vi "SubVI_Resize_Grayscale_Image #.vi"(5 "Image Register Name":string="untitled", 7 "Magnification":i32 min=1 max=9 step=1, 8 "Error In":errorcluster, 10 "ROI Descriptor":T2 {"Contours"."Type" items=["No Selection", "Point", "Line", "Rectangle", "Oval", "Polygon", "Freehand Region", "Annulus", "Unused2", "Unused3", "Broken Line", "Freehand Line", "Rotated Rectangle"]}, 11 "Image Src In":T1) -> (0 "Error Out":errorcluster, 1 "Image Src Out":T1, 2 "ROI Descriptor out":T2 {"Contours"."Type" items=["No Selection", "Point", "Line", "Rectangle", "Oval", "Polygon", "Freehand Region", "Annulus", "Unused2", "Unused3", "Broken Line", "Freehand Line", "Rotated Rectangle"]}, 3 "Image Dst Out":T1)   [LabVIEW 2013]
uses:
  <vilib>/vision/Image Controls.llb/IMAQ Image.ctl
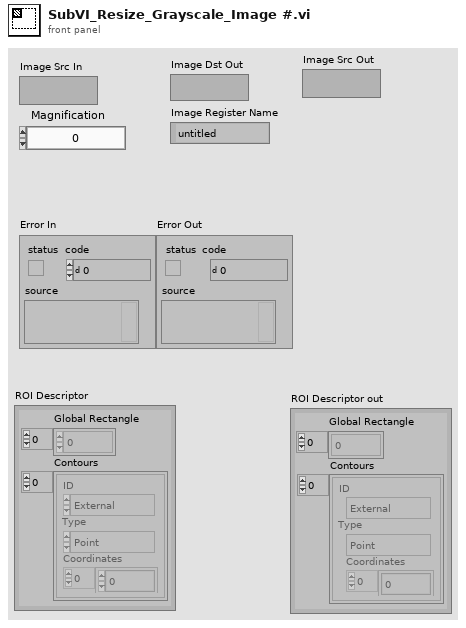
[diagram p1: front panel]
types:
  T1 = typedef "IMAQ Image.ctl" = refnum<image>
  T2 = typedef "ROI Descriptor" = cluster{"Global Rectangle":i32[], "Contours":cluster{"ID":enum32{"External", "Internal"}, "Type":u32, "Coordinates":i32[]}[]}
  T3 = enum16{"No Selection", "Point", "Line", "Rectangle", "Oval", "Polygon", "Freehand Region", "Annulus", "Unused2", "Unused3", "Broken Line", "Freehand Line", "Rotated Rectangle"}
  T4 = cluster{"ID":enum32{"External", "Internal"}, "Type":u32, "Coordinates":i32[]}[]
  T5 = cluster{"ID":enum32{"External", "Internal"}, "Type":u32, "Coordinates":i32[]}
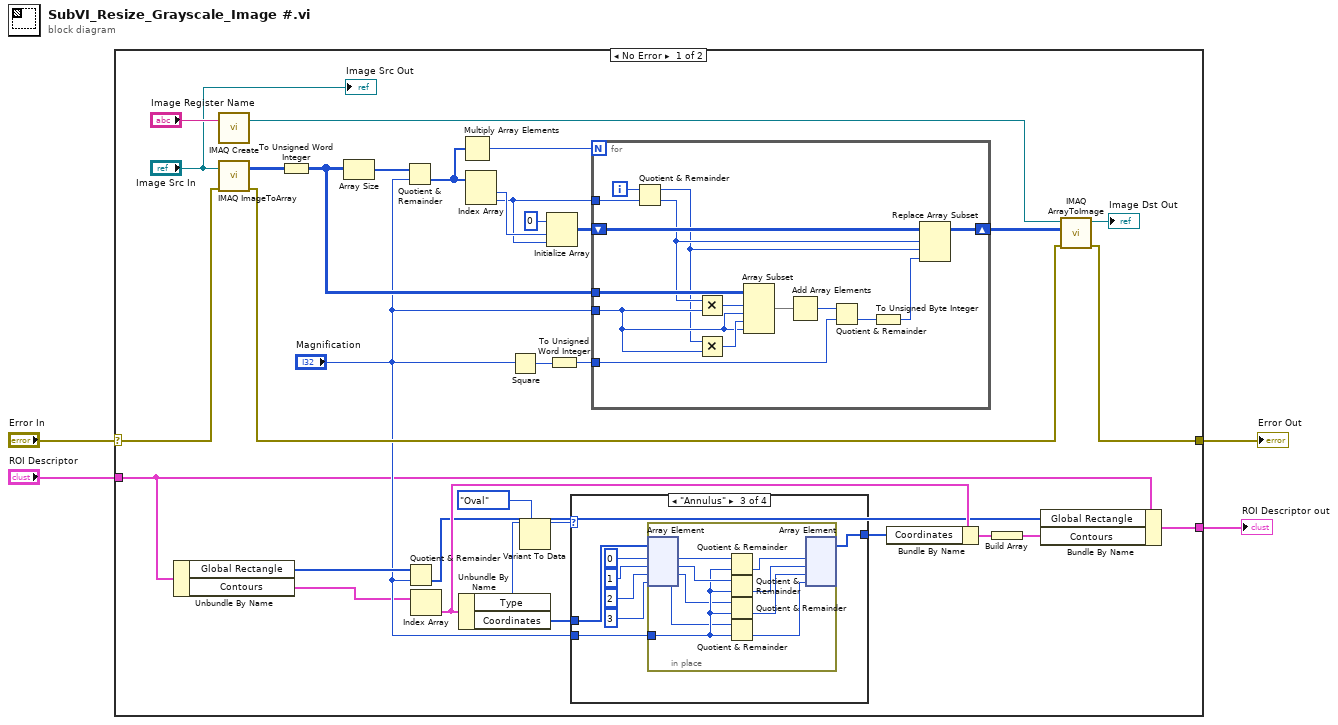
[diagram p0: block diagram]
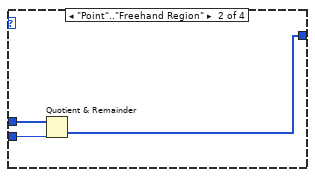
[diagram p3: hidden frame]
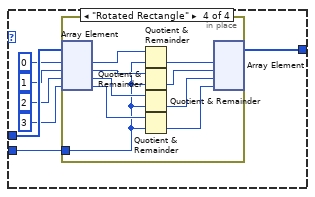
[diagram p4: hidden frame]
diagram:
  n1 = case shown="No Error" "Error In" {
    selector: "Error In" -> [w26 w90]
    tunnel: [w23 w90] -> w3
    tunnel: "ROI Descriptor" -> [w9 w89]
    tunnel: [w7 w89] -> w1
    frame No Error {
      n2 = Unbundle By Name(w9) -> ("Global Rectangle"=w19:i32[], "Contours"=w13:T4)
      n3 = call "IMAQ Create"("Image Name"="Image Register Name") -> ("New Image"=w20:T1)  [unwired: 4 in, 1 out]
      n4 = call "IMAQ ImageToArray"("error in (no error)"=w26, "Image"="Image Src In") -> ("error out"=w24:errorcluster, "Image Pixels (U8)"=w28:u8[][])  [unwired: 2 in, 3 out]
      n5 = To Unsigned Word Integer(number=w28) -> (unsigned 16bit integer=w27:u16[][])
      n6 = Array Size(array=w27) -> (size(s)=w36:i32[])
      n7 = Quotient & Remainder(x=w36, y="Magnification") -> (floor(x/y)=w37:i32[])  [unwired: 1 out]
      n8 = Quotient & Remainder(x=w19, y="Magnification") -> (floor(x/y)=w6:i32[])  [unwired: 1 out]
      n9 = Index Array(array=w13) -> (element=w12:T5)  [unwired: 1 in]
      n10 = Unbundle By Name(w12) -> ("Type"=w17:u32, "Coordinates"=w16:i32[])
      n11 = Multiply Array Elements(1:w37) -> (0:w35:i32)
      n12 = Index Array(array=w37) -> (element #1=w32:i32, element #2=w31:i32)  [unwired: 2 in]
      n13 = Square(x="Magnification") -> (x^2=w30:i32)
      n14 = Variant To Data(type=T3."Oval" ("Type"), Variant=w17) -> (data=w15:T3)  [unwired: 1 in, 1 out]
      n15 = Initialize Array(u8 0 ("element"), w32, w31) -> (w33:u8[][])
      n16 = To Unsigned Word Integer(number=w30) -> (unsigned 16bit integer=w29:u16)
      n17 = case shown="\"Annulus\"" w15 {
        tunnel: w16 -> [w38 w41 w48 w64]
        tunnel: "Magnification" -> [_ w40 w47 w63]
        tunnel: [w38 w39 w46 w62] -> w11
        frame "No Selection", Default {
        }
        frame "Point".."Freehand Region" {
          n18 = Quotient & Remainder(x=w41, y=w40) -> (floor(x/y)=w39:i32[])  [unwired: 1 out]
        }
        frame "Annulus" {
          n19 = in-place {
            in-place-border: w47 -> [w51]
            n20 = in-place-array #1(w48, 0, 1, 2, 3) -> (w57:i32, w56:i32, w50:i32, w49:i32)
            n21 = Quotient & Remainder(x=w57, y=w51) -> (floor(x/y)=w55:i32)  [unwired: 1 out]
            n22 = Quotient & Remainder(x=w56, y=w51) -> (floor(x/y)=w54:i32)  [unwired: 1 out]
            n23 = Quotient & Remainder(x=w50, y=w51) -> (floor(x/y)=w53:i32)  [unwired: 1 out]
            n24 = Quotient & Remainder(x=w49, y=w51) -> (floor(x/y)=w52:i32)  [unwired: 1 out]
            n25 = in-place-array #1(w55, w54, w53, w52) -> (w46:i32[])  [unwired: 4 out]
          }
        }
        frame "Rotated Rectangle" {
          n26 = in-place {
            in-place-border: w63 -> [w65]
            n27 = in-place-array #2(w64, 0, 1, 2, 3) -> (w69:i32, w68:i32, w67:i32, w66:i32)
            n28 = Quotient & Remainder(x=w69, y=w65) -> (floor(x/y)=w73:i32)  [unwired: 1 out]
            n29 = Quotient & Remainder(x=w68, y=w65) -> (floor(x/y)=w72:i32)  [unwired: 1 out]
            n30 = Quotient & Remainder(x=w67, y=w65) -> (floor(x/y)=w71:i32)  [unwired: 1 out]
            n31 = Quotient & Remainder(x=w66, y=w65) -> (floor(x/y)=w70:i32)  [unwired: 1 out]
            n32 = in-place-array #2(w73, w72, w71, w70) -> (w62:i32[])  [unwired: 4 out]
          }
        }
      }
      n33 = for {
        N: w35 -> [_]
        shift-right: [w74] -> w25
        shift-left: w33 -> [w78]
        tunnel: w31 -> [w87]
        tunnel: w27 -> [w81]
        tunnel: w29 -> [w80]
        tunnel: "Magnification" -> [w79]
        i -> [w88]
        n34 = Quotient & Remainder(x=w88, y=w87) -> (x-y*floor(x/y)=w75:i32, floor(x/y)=w76:i32)
        n35 = Multiply(x=w76, y=w79) -> (x*y=w83:i32)
        n36 = Multiply(x=w75, y=w79) -> (x*y=w84:i32)
        n37 = Array Subset(array=w81, index (row)=w83, length (row)=w79, index (col)=w84, length (col)=w79) -> (w82:u16[][])
        n38 = Add Array Elements(numeric array=w82) -> (sum=w86:u16)
        n39 = Quotient & Remainder(x=w86, y=w80) -> (floor(x/y)=w85:u16)  [unwired: 1 out]
        n40 = To Unsigned Byte Integer(number=w85) -> (unsigned 8bit integer=w77:u8)
        n41 = Replace Array Subset(array=w78, new element=w77, index (row)=w76, index (col)=w75) -> (w74:u8[][])
      }
      n42 = Bundle By Name(cluster=w12, "Coordinates"=w11) -> (w10:T5)
      n43 = Build Array(w10) -> (w8:T4)
      n44 = Bundle By Name(cluster=w9, "Global Rectangle"=w6, "Contours"=w8) -> (w7:T2)
      n45 = call "IMAQ ArrayToImage"("error in (no error)"=w24, "Image Pixels (U8)"=w25, "Image"=w20) -> ("error out"=w23:errorcluster, "Image Out"=→"Image Dst Out":T1)  [unwired: 7 in]
      "Image Src Out" <- "Image Src In"
    }
    frame Error {
    }
  }
  "Error Out" <- w3
  "ROI Descriptor out" <- w1
